vi "Decode Channels from Payload Data.vi"(9 "offset bytes (16)":i32=16, 10 "Parameters":T2(array[cluster]) {"encoding" items=["BNR", "BCD", "Discrete", "Signed_32", "Signed_64", "Float_32", "Float_64", "Opaque"]}, 11 "Message Buffer in":u8[](array[numeric])) -> (2 "Channels":dbl[](array[numeric]), 3 "Message Buffer out":u8[](array[numeric]))   [LabVIEW 2024]
uses:
  Encoding (Arinc664).ctl
  5ce4c490-6d47-4ac3-889b-dfcf7edbc9d5.vi
  83f7162d-6a38-4db4-a074-53e6bbb12d08.vi
  af534b45-90f6-4703-9823-abb869043907.vi
  3111cd93-0293-4347-9d69-9e92024aa7da.vi
  fed52124-c373-47e9-b8e7-95d53306dde0.vi
  459d007d-106f-4577-9e19-63051c820508.vi
  12872b70-15eb-4980-a14e-7325723023e3.vi
  5ce4c490-6d47-4ac3-889b-dfcf7edbc9d5.vi/16a2565b-3c16-407b-a626-9da2a3da432e.vi
  83f7162d-6a38-4db4-a074-53e6bbb12d08.vi/0a001d06-2809-4638-8d0b-e017d2157007.vi
  83f7162d-6a38-4db4-a074-53e6bbb12d08.vi/e08d08e5-79bf-42ec-a5e5-c4db927cd1a5.vi
  <vilib>/NI/NI VeriStand Encoding and Decoding/Get Bits Per Digit from Base.vi
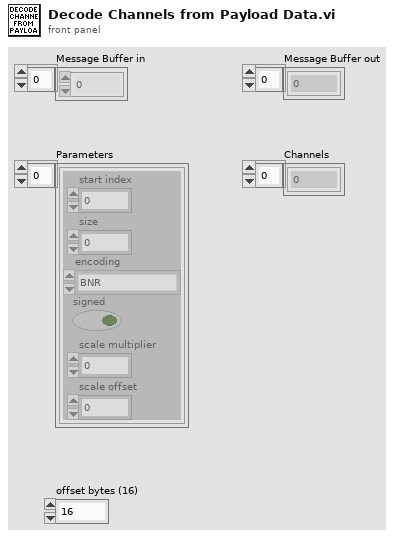
[diagram p1: front panel]
types:
  T1 = typedef "Encoding (Arinc664).ctl" = u16
  T2 = cluster{"start index":i32, "size":i32, "encoding":T1, "signed":bool, "scale multiplier":dbl, "scale offset":dbl}[]
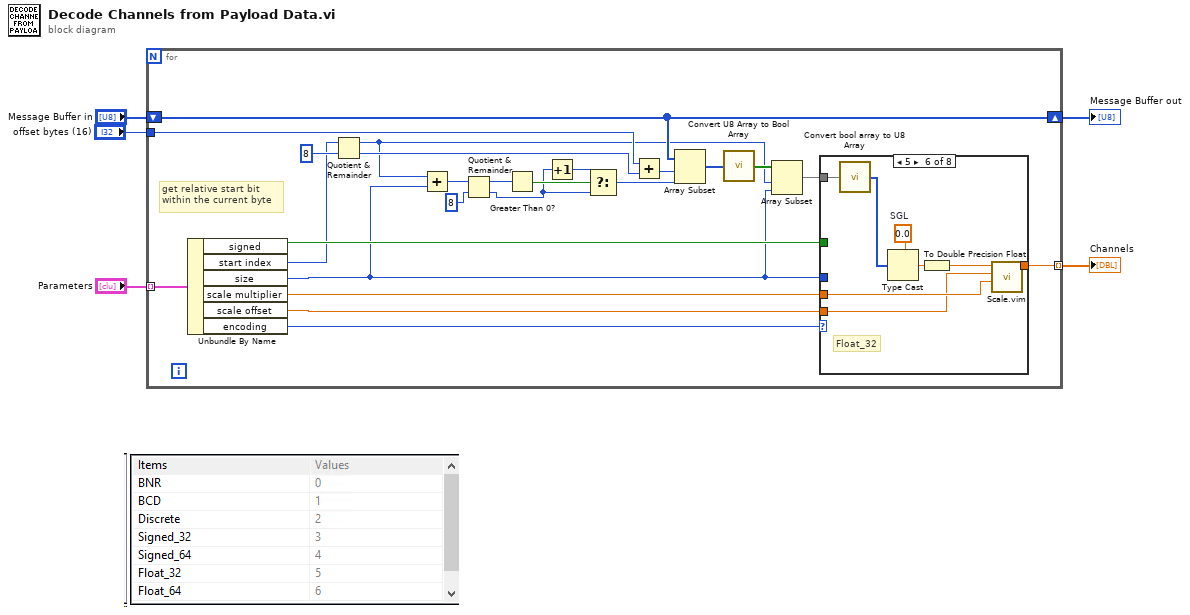
[diagram p0: block diagram]
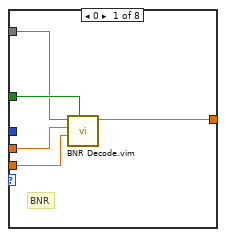
[diagram p2: hidden frame]
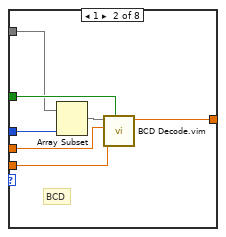
[diagram p3: hidden frame]
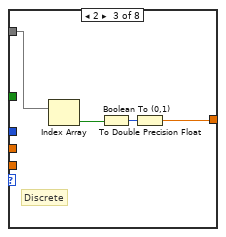
[diagram p4: hidden frame]
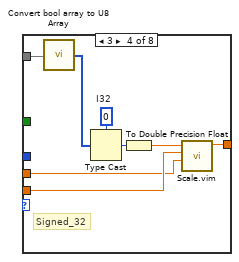
[diagram p5: hidden frame]
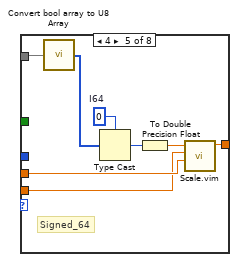
[diagram p6: hidden frame]
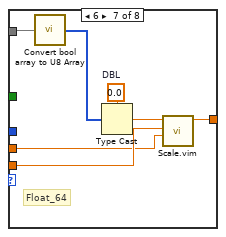
[diagram p7: hidden frame]
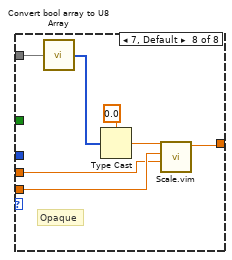
[diagram p8: hidden frame]
diagram:
  n1 = for {
    tunnel: "Parameters" -> [w29] mode=indexing
    tunnel: [w25] -> w5 mode=indexing
    tunnel: "offset bytes (16)" -> [w12]
    shift-right: [w7] -> w3
    shift-left: "Message Buffer in" -> [w7]
    # "get relative start bit \nwithin the current byte"
    n2 = Unbundle By Name(w29) -> ("signed"=w24:bool, "start index"=w16:i32, "size"=w9:i32, "scale multiplier"=w27:dbl, "scale offset"=w26:dbl, "encoding"=w28:T1)
    n3 = Quotient & Remainder(x=w16, y=8) -> (x-y*floor(x/y)=w6:i32, floor(x/y)=w13:i32)
    n4 = Add(x=w6, y=w9) -> (x+y=w23:i32)
    n5 = Quotient & Remainder(x=w23, y=8) -> (x-y*floor(x/y)=w22:i32, floor(x/y)=w20:i32)
    n6 = Greater Than 0?(x=w22) -> (x > 0?=w21:bool)
    n7 = Increment(x=w20) -> (x+1=w19:i32)
    n8 = Select(t=w19, s=w21, f=w20) -> (s? t:f=w15:i32)
    n9 = Add(x=w12, y=w13) -> (x+y=w14:i32)
    n10 = Array Subset(array=w7, index=w14, length=w15) -> (w11:u8[])
    n11 = call "Convert U8 Array to Bool Array.vi"("U8 array in"=w11) -> ("Boolean array out"=w10:bool[])  [unwired: 14 in]
    n12 = Array Subset(array=w10, index=w6, length=w9) -> (w8:bool[])
    n13 = case shown="5" w28 {
      tunnel: w24 -> [w34 w39 _ _ _ _ _ _]
      tunnel: w27 -> [w32 w40 _ w48 w57 w65 w74 w79]
      tunnel: w26 -> [w31 w37 _ w49 w56 w64 w75 w80]
      tunnel: w9 -> [_ w41 _ _ _ _ _ _]
      tunnel: [w33 w36 w42 w50 w58 w66 w72 w81] -> w25
      tunnel: w8 -> [w30 w35 w43 w47 w55 w63 w71 w78]
      frame 0 {
        # "BNR"
        n14 = call "BNR Decode.vim"("signed"=w34, "scale offset"=w31, "scale multiplier"=w32, "BNR encoded value"=w30) -> ("value"=w33:dbl)  [unwired: 7 in]
      }
      frame 1 {
        # "BCD"
        n15 = Array Subset(array=w35, length=w41) -> (w38:bool[])  [unwired: 1 in]
        n16 = call "BCD Decode.vim"("signed"=w39, "scale offset"=w37, "scale multiplier"=w40, "BCD encoded value"=w38) -> ("value"=w36:dbl)  [unwired: 7 in]
      }
      frame 2 {
        # "Discrete"
        n17 = Index Array(array=w43) -> (element=w44:bool)  [unwired: 1 in]
        n18 = Boolean To (0,1)(Boolean=w44) -> (0, 1=w45:i16)
        n19 = To Double Precision Float(number=w45) -> (double precision float=w42:dbl)
      }
      frame 3 {
        w53 = 0  # I32
        # "Signed_32"
        n20 = call "Convert bool array to U8 Array.vi"("Boolean array"=w47) -> ("Array"=w46:u8[])  [unwired: 14 in]
        n21 = Type Cast(type=w53, x=w46) -> (*(type *) &x=w52:i32)
        n22 = To Double Precision Float(number=w52) -> (double precision float=w51:dbl)
        n23 = call "Scale.vim"("scale multiplier"=w48, "scale offset"=w49, "value"=w51) -> ("scaled value"=w50:dbl)  [unwired: 8 in]
      }
      frame 4 {
        w61 = i64 0  # I64
        # "Signed_64"
        n24 = call "Convert bool array to U8 Array.vi"("Boolean array"=w55) -> ("Array"=w54:u8[])  [unwired: 14 in]
        n25 = Type Cast(type=w61, x=w54) -> (*(type *) &x=w60:i64)
        n26 = To Double Precision Float(number=w60) -> (double precision float=w59:dbl)
        n27 = call "Scale.vim"("scale multiplier"=w57, "scale offset"=w56, "value"=w59) -> ("scaled value"=w58:dbl)  [unwired: 8 in]
      }
      frame 5 {
        w69 = sgl 0.0  # SGL
        # "Float_32"
        n28 = call "Convert bool array to U8 Array.vi"("Boolean array"=w63) -> ("Array"=w62:u8[])  [unwired: 14 in]
        n29 = Type Cast(type=w69, x=w62) -> (*(type *) &x=w68:sgl)
        n30 = To Double Precision Float(number=w68) -> (double precision float=w67:dbl)
        n31 = call "Scale.vim"("scale multiplier"=w65, "scale offset"=w64, "value"=w67) -> ("scaled value"=w66:dbl)  [unwired: 8 in]
      }
      frame 6 {
        w76 = 0.0  # DBL
        # "Float_64"
        n32 = call "Convert bool array to U8 Array.vi"("Boolean array"=w71) -> ("Array"=w70:u8[])  [unwired: 14 in]
        n33 = Type Cast(type=w76, x=w70) -> (*(type *) &x=w73:dbl)
        n34 = call "Scale.vim"("scale multiplier"=w74, "scale offset"=w75, "value"=w73) -> ("scaled value"=w72:dbl)  [unwired: 8 in]
      }
      frame 7, Default {
        # "Opaque"
        n35 = call "Convert bool array to U8 Array.vi"("Boolean array"=w78) -> ("Array"=w77:u8[])  [unwired: 14 in]
        n36 = Type Cast(type=0.0 ("value"), x=w77) -> (*(type *) &x=w82:dbl)
        n37 = call "Scale.vim"("scale multiplier"=w79, "scale offset"=w80, "value"=w82) -> ("scaled value"=w81:dbl)  [unwired: 8 in]
      }
    }
  }
  "Channels" <- w5
  "Message Buffer out" <- w3
